vi "dfd_Get N(z) and D(z).vi"(2 "zeros":T1[](array[typedef]), 3 "poles":T1[](array[typedef])) -> (0 "D(z)":cluster{"Di(z)":dbl[]}[](array[cluster]) {"Di(z)" format="%.2f"}, 1 "N(z)":cluster{"Ni(z)":dbl[]}[](array[cluster]) {"Ni(z)" format="%.2f"})   [LabVIEW 2017, in "NI_DigFilter_Design.lvlib"]
uses:
  <vilib>/addons/Digital Filter Design/NI_DigFilter_Design.lvlib
  <vilib>/addons/Digital Filter Design/_Objects.llb/DFD Pole-Zero.ctl
  <vilib>/addons/Digital Filter Design/NI_DigFilterLicensed.lvlib
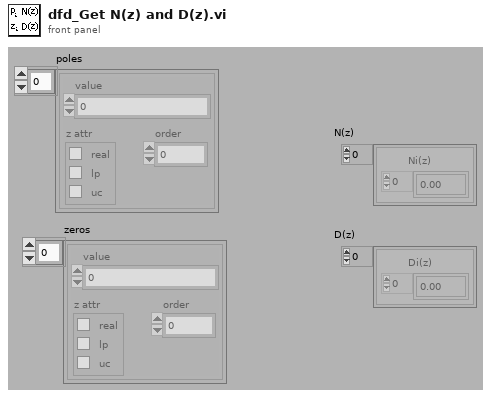
[diagram p1: front panel]
types:
  T1 = typedef "NI_DigFilterLicensed.lvlib/DFD Pole-Zero.ctl" = cluster{"value":cdb, "z attr":cluster{"real":bool, "lp":bool, "uc":bool}, "order":i32}
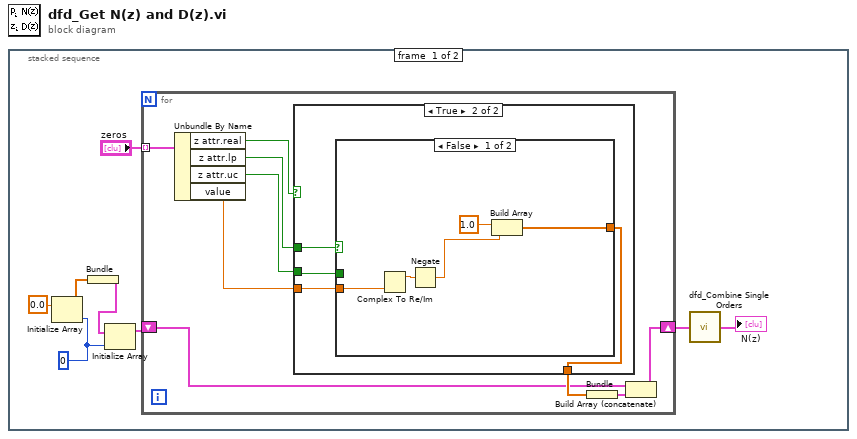
[diagram p0: block diagram]
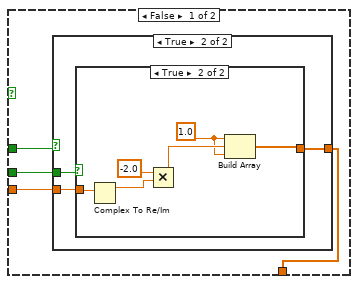
[diagram p2: hidden frame]
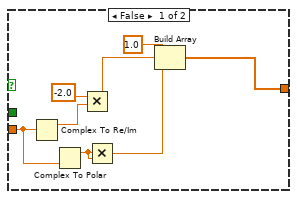
[diagram p3: hidden frame]
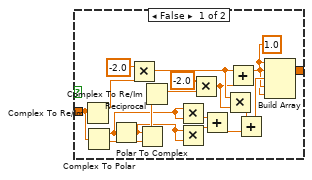
[diagram p4: hidden frame]
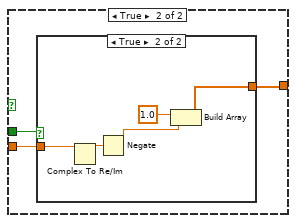
[diagram p5: hidden frame]
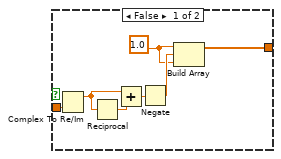
[diagram p6: hidden frame]
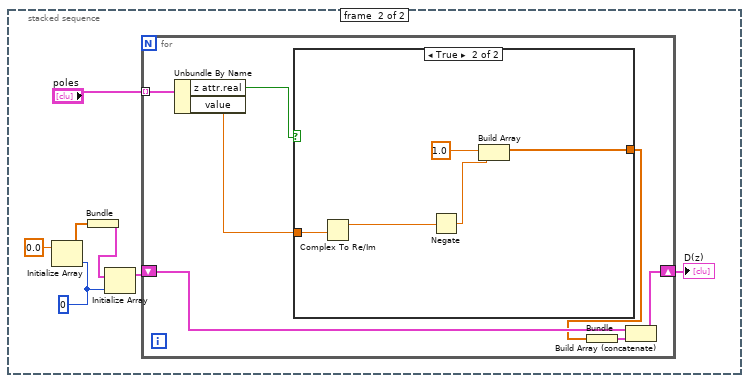
[diagram p7: hidden frame]
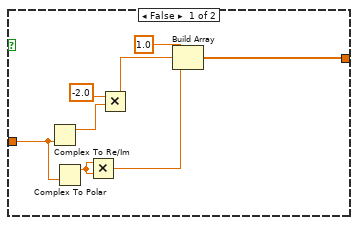
[diagram p8: hidden frame]
diagram:
  n1 = stacked-sequence {
    frame #0 {
      w3 = 0
      n2 = Initialize Array(0.0, w3) -> (w7:dbl[])
      n3 = Bundle(w7) -> (w6:cluster{dbl[]})  [unwired: 1 in]
      n4 = Initialize Array(w6, w3) -> (w5:cluster{dbl[]}[])
      n5 = for {
        tunnel: "zeros" -> [w17] mode=indexing
        shift-right: [w9] -> w4
        shift-left: w5 -> [w11]
        n6 = Unbundle By Name(w17) -> ("z attr.real"=w16:bool, "z attr.lp"=w15:bool, "z attr.uc"=w13:bool, "value"=w14:cdb)
        n7 = case shown="True" w16 {
          tunnel: w15 -> [w21 w61]
          tunnel: w14 -> [w20 w60]
          tunnel: w13 -> [w19 w58]
          tunnel: [w18 w59] -> w12
          frame False {
            n8 = case shown="True" w21 {
              tunnel: w20 -> [w26 w31]
              tunnel: [w25 w30] -> w18
              tunnel: w19 -> [_ w32]
              frame False {
                n9 = Complex To Re/Im(x + iy=w26) -> (x=w28:dbl)  [unwired: 1 out]
                n10 = Complex To Polar(r * e^(i*theta)=w26) -> (r=w24:dbl)  [unwired: 1 out]
                n11 = Multiply(x=-2.0, y=w28) -> (x*y=w27:dbl)
                n12 = Multiply(x=w24, y=w24) -> (x*y=w23:dbl)
                n13 = Build Array(1.0, w27, w23) -> (w25:dbl[])
              }
              frame True {
                n14 = case shown="True" w32 {
                  tunnel: w31 -> [w49 w52]
                  tunnel: [w33 w53] -> w30
                  frame False {
                    w34 = 1.0
                    n15 = Complex To Re/Im(x + iy=w49) -> (x=w50:dbl)  [unwired: 1 out]
                    n16 = Complex To Polar(r * e^(i*theta)=w49) -> (r=w44:dbl, theta=w48:dbl)
                    n17 = Reciprocal(x=w44) -> (1/x=w43:dbl)
                    n18 = Multiply(x=-2.0, y=w50) -> (x*y=w40:dbl)
                    n19 = Polar To Complex(1:w48, 2:w43) -> (0:w47:cdb)
                    n20 = Complex To Re/Im(x + iy=w47) -> (x=w45:dbl)  [unwired: 1 out]
                    n21 = Multiply(x=w44, y=w44) -> (x*y=w42:dbl)
                    n22 = Multiply(x=w43, y=w43) -> (x*y=w41:dbl)
                    n23 = Multiply(x=-2.0, y=w45) -> (x*y=w39:dbl)
                    n24 = Add(x=w42, y=w41) -> (x+y=w37:dbl)
                    n25 = Multiply(x=w40, y=w39) -> (x*y=w38:dbl)
                    n26 = Add(x=w40, y=w39) -> (x+y=w35:dbl)
                    n27 = Add(x=w38, y=w37) -> (x+y=w36:dbl)
                    n28 = Build Array(w34, w35, w36, w35, w34) -> (w33:dbl[])
                  }
                  frame True {
                    w54 = 1.0
                    n29 = Complex To Re/Im(x + iy=w52) -> (x=w56:dbl)  [unwired: 1 out]
                    n30 = Multiply(x=-2.0, y=w56) -> (x*y=w55:dbl)
                    n31 = Build Array(w54, w55, w54) -> (w53:dbl[])
                  }
                }
              }
            }
          }
          frame True {
            n32 = case shown="False" w61 {
              tunnel: w60 -> [w66 w69]
              tunnel: [w64 w68] -> w59
              tunnel: w58 -> [_ w67]
              frame False {
                n33 = Complex To Re/Im(x + iy=w66) -> (x=w65:dbl)  [unwired: 1 out]
                n34 = Negate(x=w65) -> (-x=w62:dbl)
                n35 = Build Array(1.0, w62) -> (w64:dbl[])
              }
              frame True {
                n36 = case shown="True" w67 {
                  tunnel: [w76 w77] -> w68
                  tunnel: w69 -> [w70 w78]
                  frame False {
                    w71 = 1.0
                    n37 = Complex To Re/Im(x + iy=w70) -> (x=w73:dbl)  [unwired: 1 out]
                    n38 = Reciprocal(x=w73) -> (1/x=w72:dbl)
                    n39 = Add(x=w73, y=w72) -> (x+y=w74:dbl)
                    n40 = Negate(x=w74) -> (-x=w75:dbl)
                    n41 = Build Array(w71, w75, w71) -> (w76:dbl[])
                  }
                  frame True {
                    n42 = Complex To Re/Im(x + iy=w78) -> (x=w81:dbl)  [unwired: 1 out]
                    n43 = Negate(x=w81) -> (-x=w79:dbl)
                    n44 = Build Array(1.0, w79) -> (w77:dbl[])
                  }
                }
              }
            }
          }
        }
        n45 = Bundle(w12) -> (w10:cluster{dbl[]})  [unwired: 1 in]
        n46 = Build Array (concatenate)(w11, w10) -> (w9:cluster{dbl[]}[])
      }
      n47 = call <vilib>:"dfd_Combine Single Orders.vi"("P(z) in"=w4) -> ("P(z) out"=→"N(z)":cluster{"Ni(z)":dbl[]}[])
    }
    frame #1 {
      w85 = 0
      n48 = Initialize Array(0.0, w85) -> (w88:dbl[])
      n49 = Bundle(w88) -> (w87:cluster{dbl[]})  [unwired: 1 in]
      n50 = Initialize Array(w87, w85) -> (w86:cluster{dbl[]}[])
      n51 = for {
        tunnel: "poles" -> [w95] mode=indexing
        shift-right: [w90] -> w82
        shift-left: w86 -> [w92]
        n52 = Unbundle By Name(w95) -> ("z attr.real"=w94:bool, "value"=w93:cdb)
        n53 = case shown="True" w94 {
          tunnel: w93 -> [w98 w107]
          tunnel: [w100 w108] -> w89
          frame False {
            n54 = Complex To Re/Im(x + iy=w98) -> (x=w102:dbl)  [unwired: 1 out]
            n55 = Complex To Polar(r * e^(i*theta)=w98) -> (r=w99:dbl)  [unwired: 1 out]
            n56 = Multiply(x=w99, y=w99) -> (x*y=w96:dbl)
            n57 = Multiply(x=-2.0, y=w102) -> (x*y=w101:dbl)
            n58 = Build Array(1.0, w101, w96) -> (w100:dbl[])
          }
          frame True {
            n59 = Complex To Re/Im(x + iy=w107) -> (x=w106:dbl)  [unwired: 1 out]
            n60 = Negate(x=w106) -> (-x=w104:dbl)
            n61 = Build Array(1.0, w104) -> (w108:dbl[])
          }
        }
        n62 = Bundle(w89) -> (w91:cluster{dbl[]})  [unwired: 1 in]
        n63 = Build Array (concatenate)(w92, w91) -> (w90:cluster{dbl[]}[])
      }
      "D(z)" <- w82
    }
  }
